vi "URL(subVI).vi"() -> (2 "URL":string="https://27bhujjo.pp.vuforia.io:8443/Thingworx/Things/NI.cRIO.DemoKit/Services/crioEndpoint?postParameter=json ")   [LabVIEW 2017]
panel:
  in  "Boolean":bool
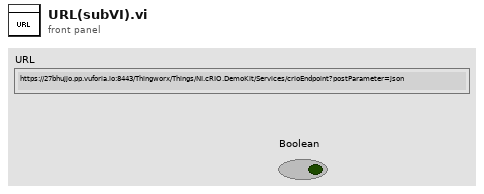
[diagram p1: front panel]
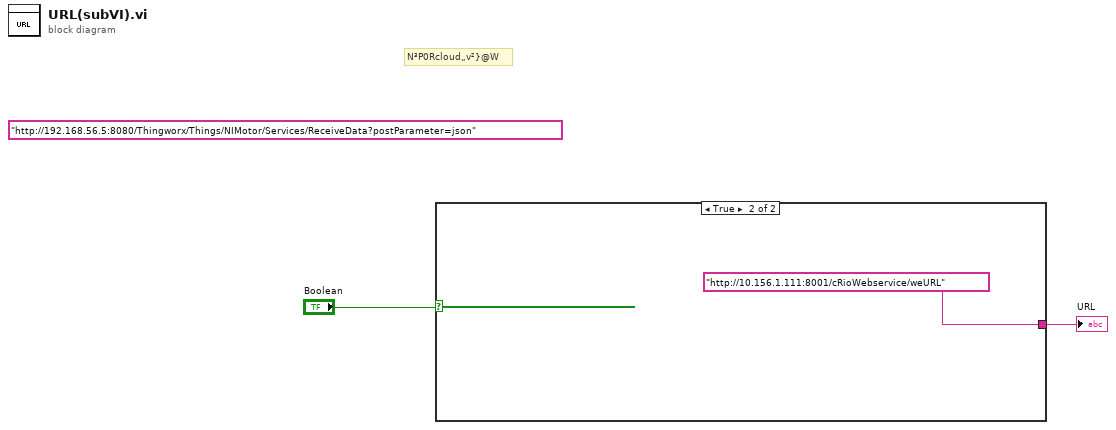
[diagram p0: block diagram]
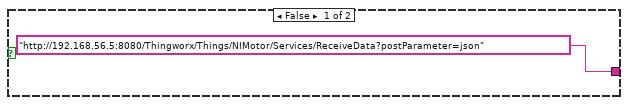
[diagram p2: hidden frame]
diagram:
  (unwired) "http://192.168.56.5:8080/Thingworx/Things/NIMotor/Services/ReceiveData?postParameter=json"
  # "N³P0Rcloud„v²}@W"
  n1 = case shown="True" "Boolean" {
    tunnel: ["http://192.168.56.5:8080/Thingworx/Things/NIMotor/Services/ReceiveData?postParameter=json" "http://10.156.1.111:8001/cRioWebservice/weURL"] -> w1
    frame False {
    }
    frame True {
    }
  }
  "URL" <- w1
